vi "LaunchUI.vi"() -> ()   [LabVIEW 2019]
uses:
  Components/ViPER.lvlibp/ViPER.lvclass
panel:
  out "error out":errorcluster
  in  "String":string="<Object><Name>MES</Name><Class>MES_Local</Class><Config><NumElts>1</NumElts><Path><Name>Results_Path</Name><Val>C:\\Nanosonics</Val></Path></Config><Objects><Object><Name>Login</Name><Class>Login_Dialog</Class><Config><NumElts>1</NumElts><String><Name>default</Name><Val /></String></Config><Ancestors><Ancestor><Class>Login_Base</Class><Config><NumElts>1</NumElts><String><Name>default</Name><Val /></String></Config></Ancestor></Ancestors></Object></Objects><Ancestors><Ancestor><Class>MES_Base</Class><Config><NumElts>1</NumElts><String><Name>WorkflowStep</Name><Val>P5_PCB</Val></String></Config></Ancestor></Ancestors></Object>"
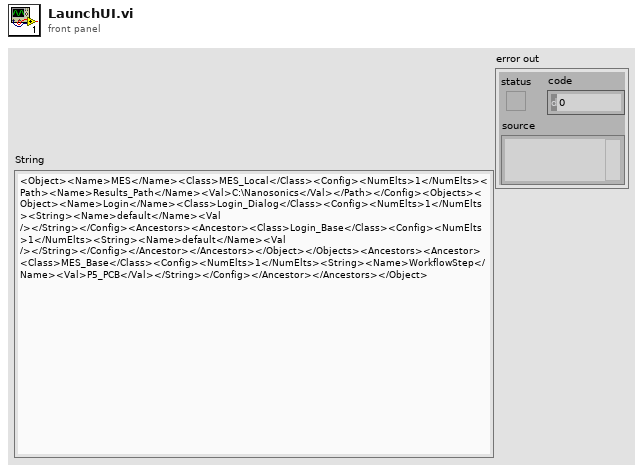
[diagram p1: front panel]
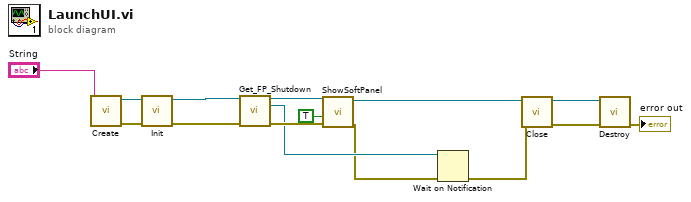
[diagram p0: block diagram]
diagram:
  n1 = call "Create.vi"("Config XML"="String") -> ("error out"=w13:errorcluster, "reference out"=w14:refnum<class "ViPER.lvclass">)  [unwired: 9 in]
  n2 = call-dynamic "Init.vi"("error in (no error)"=w13, "reference in"=w14) -> ("error out"=w11:errorcluster, "reference out"=w12:refnum<class "ViPER.lvclass">)  [unwired: 8 in]
  n3 = call "Get_FP_Shutdown.vi"("ViKing_Base in"=w12, "error in (no error)"=w11) -> ("ViKing_Base out"=w10:refnum<class "ViPER.lvclass">, "SoftFP_Shutdown"=w8:refnum<notifier>, "error out"=w9:errorcluster)  [unwired: 9 in, 2 out]
  n4 = call-dynamic "ShowSoftPanel.vi"("error in (no error)"=w9, "Floating"=TRUE, "Driver in"=w10) -> ("error out"=w7:errorcluster, "Driver out"=w4:refnum<class "ViPER.lvclass">)  [unwired: 6 in, 1 out]
  n5 = Wait on Notification(notifier=w8, error in (no error)=w7) -> (error out=w5:errorcluster)  [unwired: 2 in, 3 out]
  n6 = call-dynamic "Close.vi"("error in (no error)"=w5, "reference in"=w4) -> ("error out"=w3:errorcluster, "reference out"=w2:refnum<class "ViPER.lvclass">)  [unwired: 8 in]
  n7 = call "Destroy.vi"("error in (no error)"=w3, "reference in"=w2) -> ("error out"=→"error out":errorcluster)  [unwired: 9 in]
